vi "OnPercentComplete Event Callback.vi"(4 "Percent Complete Message":refnum<user-event>, 5 "Event Data":cluster{"percent":dbl}, 6 "Control Ref":refnum<k24>, 7 "Event Common Data":T1) -> ()   [LabVIEW 2020, in "NI_VS MacroPlayerAPI.lvlib"]
uses:
  <vilib>/NI VeriStand/Execution/MacroPlayer/NI_VS MacroPlayerAPI.lvlib
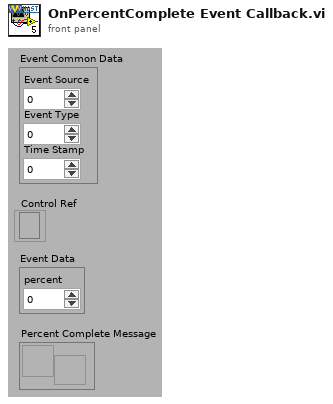
[diagram p1: front panel]
types:
  T1 = cluster{"Event Source":i32, "Event Type":u32, "Time Stamp":u32}
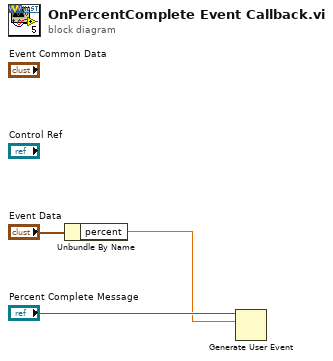
[diagram p0: block diagram]
diagram:
  n1 = Unbundle By Name("Event Data") -> ("percent"=w1:dbl)
  n2 = Generate User Event(user event="Percent Complete Message", event data cluster=w1) -> ()  [unwired: 2 in, 2 out]
